vi "StopRecord.vi"(8 "error in (no error)":errorcluster, 10 "Label":string, 11 "Task_Abstr in":refnum<class "Task_Abstr.lvclass">) -> (0 "error out":errorcluster, 3 "Task_Abstr out":refnum<class "Task_Abstr.lvclass">)   [LabVIEW 2025, in "Task_Abstr.lvlib" / "Task_Abstr.lvclass"]
uses:
  Task_Abstr.lvclass
  Task_Abstr.lvclass/Task_Abstr.ctl
  <vilib>/Utility/miscctls.llb/LVMapReplaceAction.ctl
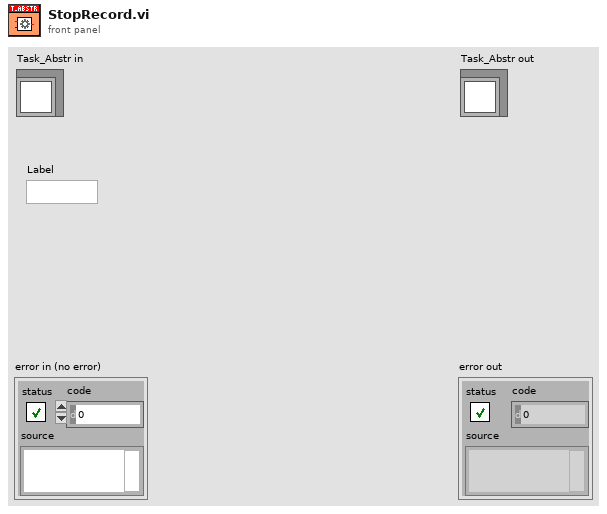
[diagram p1: front panel]
types:
  T1 = typedef "LVMapReplaceAction.ctl" = enum32{"Modify Entry only if found", "Add or Modify Entry", "Delete Entry"}
  T2 = typedef "Task_Abstr.lvlib/Task_Abstr.lvclass/DataContainer.ctl" = map{string, T3}
  T3 = typedef "Task_Abstr.lvlib/Task_Abstr.lvclass/WaveformData.ctl" = cluster{"StartTime":timestamp, "StopTime":timestamp, "Waveform":waveform(dbl)[]}
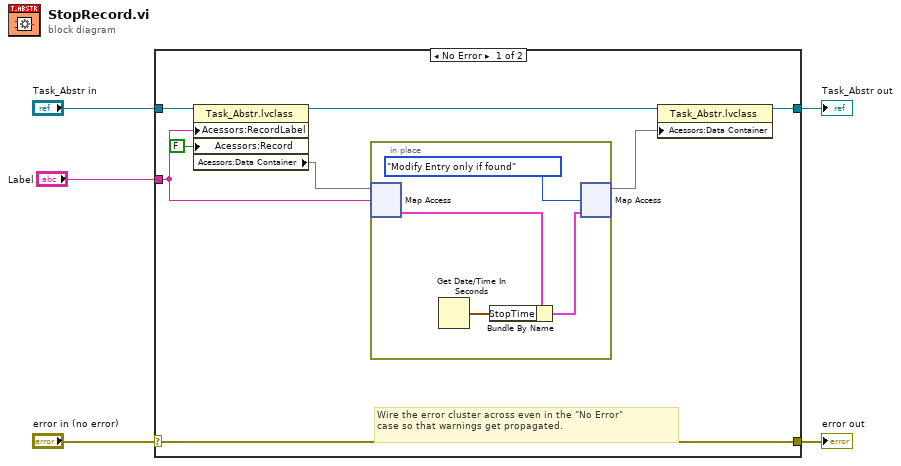
[diagram p0: block diagram]
diagram:
  n1 = case shown="No Error" "error in (no error)" {
    selector: "error in (no error)" -> [w13 w19]
    tunnel: [w13 w19] -> w4
    tunnel: [w8 w18] -> w2
    tunnel: "Task_Abstr in" -> [w9 w18]
    tunnel: "Label" -> [w6 _]
    frame No Error {
      # "Wire the error cluster across even in the \"No Error\"\ncase so that warnings get propagated."
      n2 = property class="Task_Abstr.lvclass"(reference=w9, "Acessors:RecordLabel"=w6, "Acessors:Record"=FALSE ("Record")) -> (reference out=w12:refnum<class "Task_Abstr.lvclass">, "Acessors:Data Container"=w11:T2)  [unwired: 1 in, 1 out]
      n3 = in-place {
        n4 = in-place-map #1(w11, w6) -> (w14:T3)  [unwired: 1 in, 1 out]
        n5 = Get Date/Time In Seconds() -> (seconds since 1Jan1904=w15:timestamp)
        n6 = Bundle By Name(cluster=w14, "StopTime"=w15) -> (w16:T3)
        n7 = in-place-map #1(w16, LVMapReplaceAction."Modify Entry only if found" ("action")) -> (w10:T2)  [unwired: 2 out]
      }
      n8 = property class="Task_Abstr.lvclass"(reference=w12, "Acessors:Data Container"=w10) -> (reference out=w8:refnum<class "Task_Abstr.lvclass">)  [unwired: 1 in, 1 out]
    }
    frame Error {
    }
  }
  "error out" <- w4
  "Task_Abstr out" <- w2
